vi "SSL_free.vi"(8 "error in (no error)":errorcluster, 11 "SSL in":refnum<class "SSL.lvclass">) -> (0 "error out":errorcluster)   [LabVIEW 2013, in "OpenSSL Socket.lvlib" / "SSL.lvclass"]
uses:
  SSL.lvclass
  SSL-Lib/SSL-Lib.lvclass/SSL-Lib.ctl
  SSL.lvclass/SSL.ctl
  SSL-Lib/Read SSL Library Path.vi
  Read Handle.vi
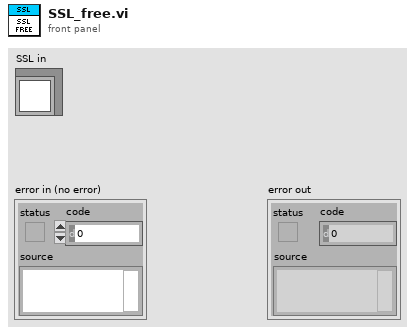
[diagram p1: front panel]
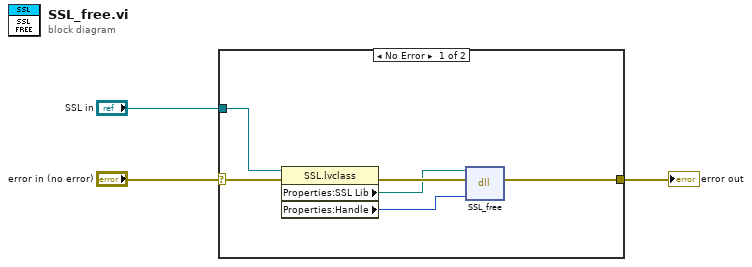
[diagram p0: block diagram]
diagram:
  n1 = case shown="No Error" "error in (no error)" {
    selector: "error in (no error)" -> [w9 w10]
    tunnel: [w8 w10] -> w2
    tunnel: "SSL in" -> [w6 _]
    frame No Error {
      n2 = property class="SSL.lvclass"(reference=w6, error in=w9) -> (error out=w7:errorcluster, "Properties:SSL Lib"=w5:path, "Properties:Handle"=w4:u64)  [unwired: 1 out]
      n3 = dll-call lib="C:/Program Files (x86)/National Instruments/Shared/nissl/NIssleay32.dll" fn="SSL_free"(path in=w5, error in=w7, "*SSL"=w4) -> (error out=w8:errorcluster)  [unwired: 3 in, 1 out]
    }
    frame Error {
    }
  }
  "error out" <- w2
